vi "DEV Get Hardware Info.vi"(10 "pHardwareInfo":T1, 11 "DevHandle":i32) -> (2 "pHardwareInfo out":T1, 3 "function return":u8)   [LabVIEW 2010, in "usb_device.lvlib"]
doc: "unsigned char WINAPI DEV_GetHardwareInfo(int DevHandle, HARDWARE_INFO *pHardwareInfo);"
uses:
  usb_device.lvlib
  USB2XXX/trunk/USB2XXX/USB2XXX/vs2019/Release/USB2XXX.dll
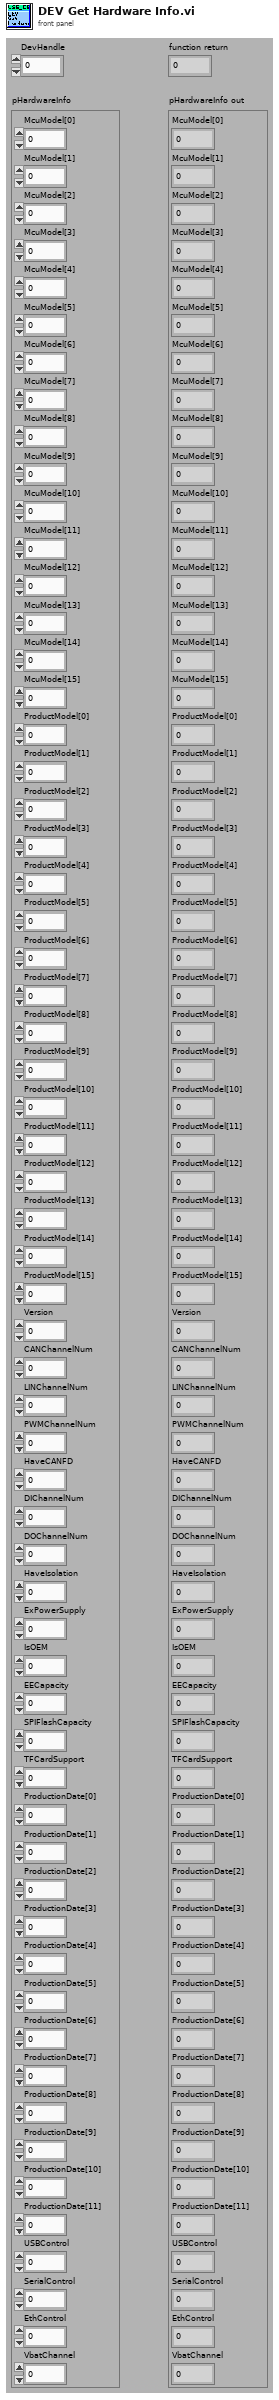
[diagram p1: front panel]
types:
  T1 = cluster{"McuModel[0]":u8, "McuModel[1]":u8, "McuModel[2]":u8, "McuModel[3]":u8, "McuModel[4]":u8, "McuModel[5]":u8, "McuModel[6]":u8, "McuModel[7]":u8, "McuModel[8]":u8, "McuModel[9]":u8, "McuModel[10]":u8, "McuModel[11]":u8, "McuModel[12]":u8, "McuModel[13]":u8, "McuModel[14]":u8, "McuModel[15]":u8, "ProductModel[0]":u8, "ProductModel[1]":u8, "ProductModel[2]":u8, "ProductModel[3]":u8, "ProductModel[4]":u8, "ProductModel[5]":u8, "ProductModel[6]":u8, "ProductModel[7]":u8, "ProductModel[8]":u8, "ProductModel[9]":u8, "ProductModel[10]":u8, "ProductModel[11]":u8, "ProductModel[12]":u8, "ProductModel[13]":u8, "ProductModel[14]":u8, "ProductModel[15]":u8, "Version":u32, "CANChannelNum":u8, "LINChannelNum":u8, "PWMChannelNum":u8, "HaveCANFD":u8, "DIChannelNum":u8, "DOChannelNum":u8, "HaveIsolation":u8, "ExPowerSupply":u8, "IsOEM":u8, "EECapacity":u8, "SPIFlashCapacity":u8, "TFCardSupport":u8, "ProductionDate[0]":u8, "ProductionDate[1]":u8, "ProductionDate[2]":u8, "ProductionDate[3]":u8, "ProductionDate[4]":u8, "ProductionDate[5]":u8, "ProductionDate[6]":u8, "ProductionDate[7]":u8, "ProductionDate[8]":u8, "ProductionDate[9]":u8, "ProductionDate[10]":u8, "ProductionDate[11]":u8, "USBControl":u8, "SerialControl":u8, "EthControl":u8, "VbatChannel":u8}
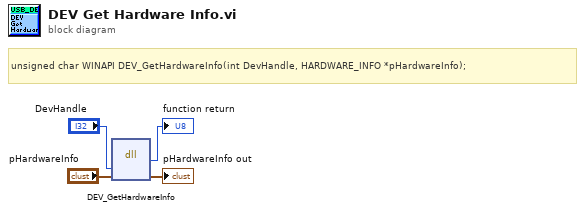
[diagram p0: block diagram]
diagram:
  # "unsigned char WINAPI DEV_GetHardwareInfo(int DevHandle, HARDWARE_INFO *pHardwareInfo);"
  n1 = dll-call lib="E:/Projects/USB2XXX/trunk/USB2XXX/USB2XXX/vs2019/Release/USB2XXX.*" fn="DEV_GetHardwareInfo"("DevHandle"="DevHandle", "pHardwareInfo"="pHardwareInfo") -> (→"function return":u8, "pHardwareInfo"=→"pHardwareInfo out":T1)  [unwired: 4 in, 2 out]
